vi "write.vi"(8 "error in (no error)":errorcluster caption="错误输入（无错误）", 10 "write":string, 11 "serial 输入":refnum<class "serial.lvclass">) -> (0 "error out":errorcluster caption="错误输出", 3 "serial 输出":refnum<class "serial.lvclass">)   [LabVIEW 2016, in "潮位站数据传输.lvlib" / "serial.lvclass"]
uses:
  serial.lvclass
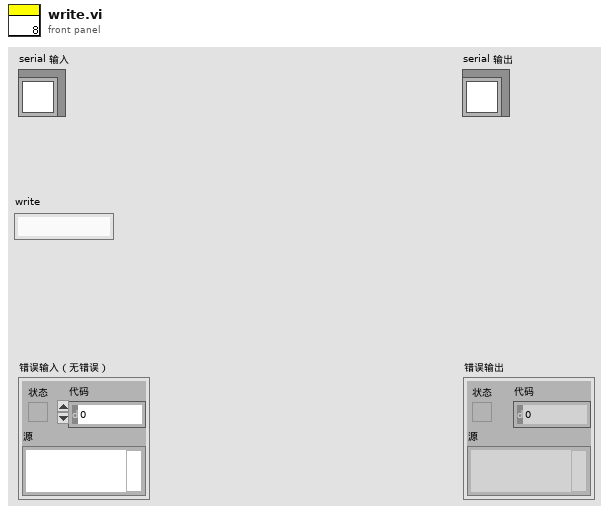
[diagram p1: front panel]
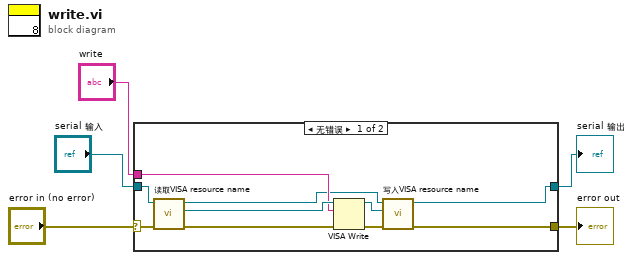
[diagram p0: block diagram]
diagram:
  n1 = case shown="无错误" "error in (no error)" {
    selector: "error in (no error)" -> [w14 w16]
    tunnel: "serial 输入" -> [w15 w17]
    tunnel: "write" -> [w12 _]
    tunnel: [w8 w17] -> w2
    tunnel: [w6 w16] -> w1
    frame No Error {
      n2 = call-dynamic "读取VISA resource name.vi"("error in (no error)"=w14, "data_inter输入"=w15) -> ("error out"=w11:errorcluster, "VISA resource name"=w13:refnum<visa-resource-name>, "data_inter输出"=w10:refnum<class "serial.lvclass">)  [unwired: 7 in]
      n3 = VISA Write(VISA resource name=w13, write buffer=w12, error in (no error)=w11) -> (VISA resource name out=w9:refnum<visa-resource-name>, error out=w7:errorcluster)  [unwired: 1 out]
      n4 = call-dynamic "写入VISA resource name.vi"("error in (no error)"=w7, "VISA resource name"=w9, "data_inter输入"=w10) -> ("error out"=w6:errorcluster, "data_inter输出"=w8:refnum<class "serial.lvclass">)  [unwired: 7 in]
    }
    frame Error {
    }
  }
  "error out" <- w1
  "serial 输出" <- w2
